vi "总圈数判定11.vi"(0 "总圈数":sgl, 1 "总圈数":cluster{"下限":dbl, "上限":dbl}, 3 "错误输入":errorcluster) -> (8 "OK":bool, 10 "错误输出":errorcluster)   [LabVIEW 2018]
uses:
  Global_Variable/Global.vi
  Global_Variable/A180648.vi
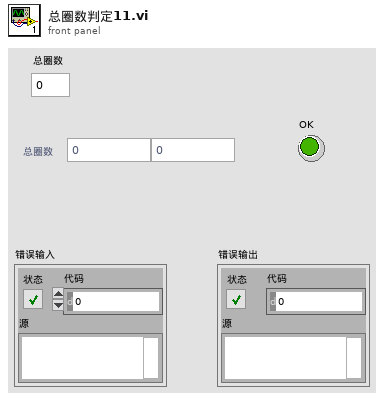
[diagram p1: front panel]
types:
  T1 = enum32{"空载", "功能", "力特性", "传感器特性", "电流特性", "振动NVH", "逆向空载", "完成"}
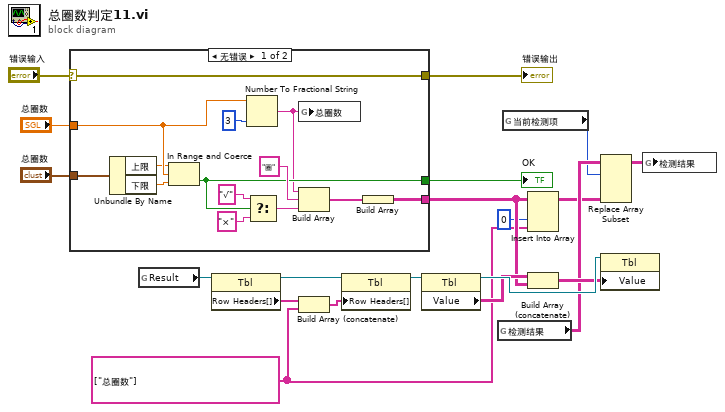
[diagram p0: block diagram]
diagram:
  w2 = string[] ["总圈数"] ("元素")
  n1 = case shown="无错误" "错误输入" {
    selector: "错误输入" -> [w27 w35]
    tunnel: [w27 w35] -> w19
    tunnel: [w29 _] -> w4
    tunnel: "总圈数" -> [w26 _]
    tunnel: "总圈数" -> [w25 _]
    tunnel: [w22 _] -> w8
    frame No Error {
      n2 = Unbundle By Name(w26) -> ("上限"=w24:dbl, "下限"=w23:dbl)
      n3 = In Range and Coerce(upper limit=w24, x=w25, lower limit=w23) -> (In Range?=w22:bool)  [unwired: 1 out]
      n4 = Number To Fractional String(number=w25, precision (6)=i16 3 ("精度(6)")) -> (F-format string=w21:string)  [unwired: 2 in]
      n5 = Select(t="√", s=w22, f="×") -> (s? t:f=w30:string)
      n6 = global write "检测结果.vi" "总圈数"(w21) -> ()
      n7 = Build Array(w21, "圈" ("元素"), w30) -> (w28:string[])
      n8 = Build Array(w28) -> (w29:string[][])
    }
    frame Error {
    }
  }
  "错误输出" <- w19
  "OK" <- w8
  n9 = global read "Global.vi" "Result"() -> (w18:refnum<vi>)
  n10 = property class="Tbl"(reference=w18) -> (reference out=w15:refnum<vi>, "Row Headers[]"=w17:string[])  [unwired: 1 in, 1 out]
  n11 = Build Array (concatenate)(w17, w2) -> (w16:string[])
  n12 = property class="Tbl"(reference=w15, "Row Headers[]"=w16) -> (reference out=w14:refnum<vi>)  [unwired: 1 in, 1 out]
  n13 = property class="Tbl"(reference=w14) -> (reference out=w13:refnum<vi>, "Value"=w12:string[][])  [unwired: 1 in, 1 out]
  n14 = global read "A180648.vi" "检测结果"() -> (w7:string[][][])
  n15 = global read "A180648.vi" "当前检测项"() -> (w6:T1)
  n16 = Insert Into Array(array=w4, index (col)=0 ("禁用的索引 (列)"), new element=w2) -> (w1:string[][])  [unwired: 1 in]
  n17 = Build Array (concatenate)(w12, w4) -> (w11:string[][])
  n18 = Replace Array Subset(array=w7, new element=w1, index (dim 0)=w6) -> (w5:string[][][])  [unwired: 2 in]
  n19 = property class="Tbl"(reference=w13, "Value"=w11) -> ()  [unwired: 1 in, 2 out]
  n20 = global write "A180648.vi" "检测结果"(w5) -> ()
